vi "TestError.vi"() -> ()   [LabVIEW 2014, in "NISTErrorLib.lvlib"]
doc: "Use this template to build a producer/consumer design pattern with events to produce queue items. Use this design pattern instead of the User Interface Event Handler pattern for user interfaces when you want to execute code asynchronously in response to an event without slowing the user interface responsiveness."
uses:
  NISTErrorLib.lvlib
  <vilib>/Utility/error.llb/Error Cluster From Error Code.vi
  <vilib>/ErrorRing/Error Ring.xnode
panel:
  in  "btnLargeError":bool
  in  "btnLog":bool
  out "Log":string
  in  "btnMultiError":bool
  out "State":string
  in  "btnStateError":bool
  in  "btnUnhandled":bool
  in  "stop":bool
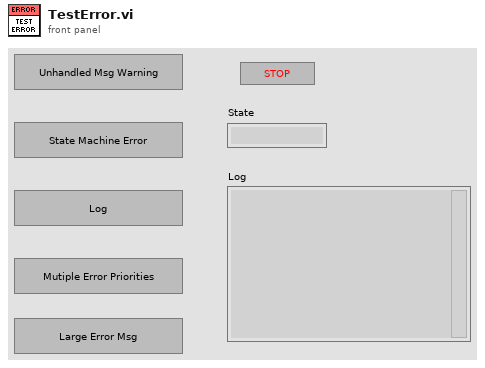
[diagram p1: front panel]
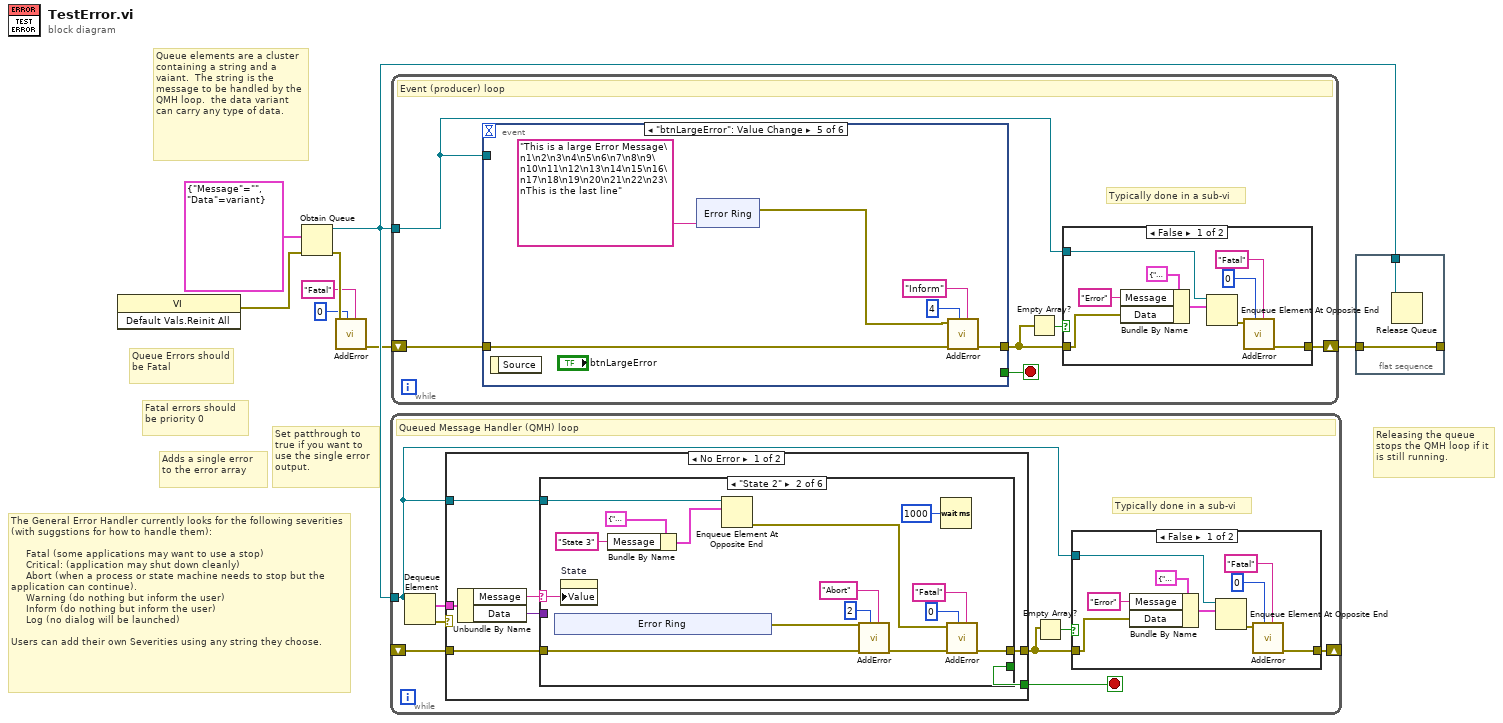
[diagram p0: block diagram]
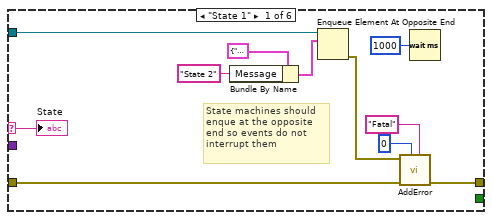
[diagram p3: hidden frame]
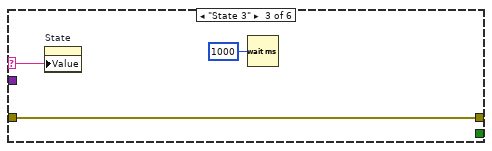
[diagram p4: hidden frame]
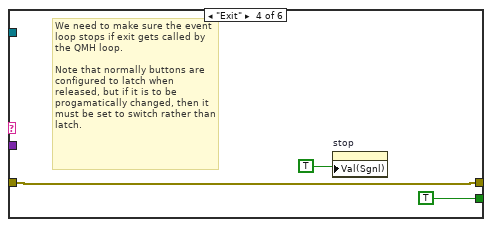
[diagram p5: hidden frame]
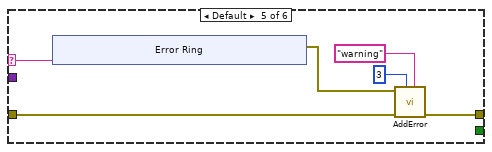
[diagram p6: hidden frame]
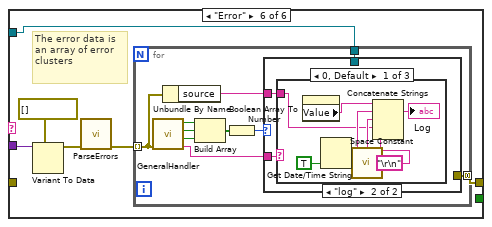
[diagram p7: hidden frame]
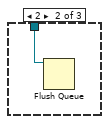
[diagram p9: hidden frame]
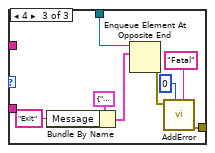
[diagram p10: hidden frame]
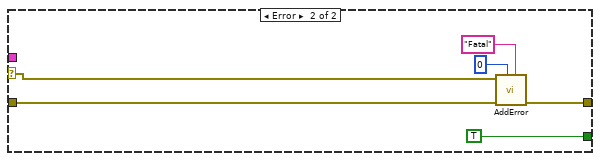
[diagram p11: hidden frame]
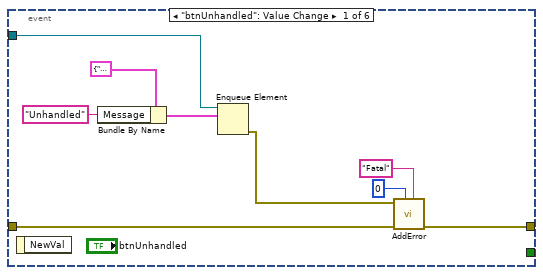
[diagram p13: hidden frame]
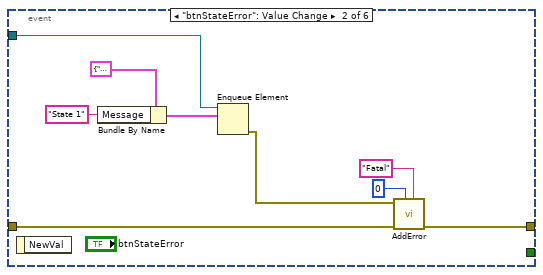
[diagram p14: hidden frame]
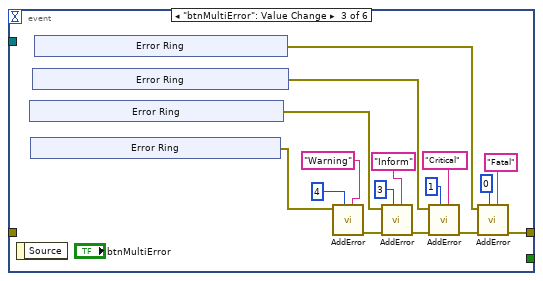
[diagram p15: hidden frame]
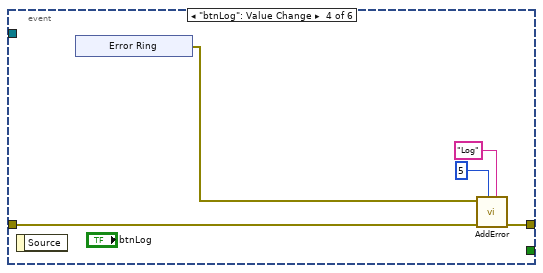
[diagram p16: hidden frame]
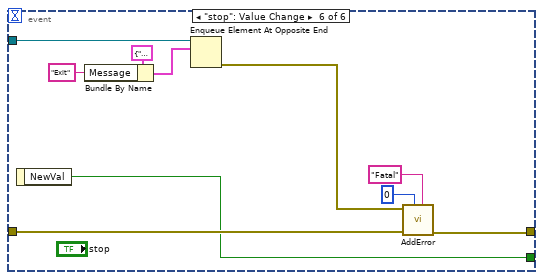
[diagram p17: hidden frame]
diagram:
  # "Set patthrough to\ntrue if you want to\nuse the single error \noutput."
  # "The General Error Handler currently looks for the following severities (with suggstions for how to handle them):\n\n     Fatal (some applications may want to use a stop)  \n     Critical: (application may shut down cleanly)\n     Abort (when a process or state machine needs to stop but the application can continue).\n     Warning (do nothing but inform the user)\n     Inform (do nothing but inform the user)\n     Log (no dialog will be launched)\n    \nUsers can add their own Severities using any string they choose."
  # "Adds a single error to the error array"
  # "Fatal errors should be priority 0"
  # "Queue elements are a cluster containing a string and a vaiant.  The string is the message to be handled by the QMH loop.  the data variant can carry any type of data."
  # "Queue Errors should be Fatal"
  # "Releasing the queue stops the QMH loop if it is still running."
  n1 = invoke class="VI" method="Default Vals.Reinit All"() -> (error out=w1:errorcluster)  [unwired: 3 in, 2 out]
  n2 = Obtain Queue(element data type=cluster{"Message":string, "Data":variant} {"Message"="", "Data"=variant}, error in (no error)=w1) -> (queue out=w8:refnum<queue>, error out=w6:errorcluster)  [unwired: 3 in, 1 out]
  n3 = call "AddError.vi"("Severity"="Fatal" ("String"), "Priority"=u8 0, "error in (no error)"=w6) -> ("ErrorArray"=w3:errorcluster[])  [unwired: 7 in, 1 out]
  n4 = while {
    tunnel: w8 -> [w11]
    shift-right: [w14] -> _
    shift-left: _ -> [w13]
    stop <- w15 stop-if-true
    # "Typically done in a sub-vi"
    # "Queued Message Handler (QMH) loop"
    n5 = Dequeue Element(queue=w11) -> (element=w12:cluster{"Message":string, "Data":variant}, error out=w16:errorcluster)  [unwired: 2 in, 2 out]
    n6 = case shown="No Error" w16 {
      selector: w16 -> [_ w120]
      tunnel: w12 -> [w33 _]
      tunnel: [w28 TRUE] -> w15
      tunnel: w13 -> [w31 w122]
      tunnel: [w30 w121] -> w10
      tunnel: w11 -> [w27 _]
      frame No Error {
        n7 = Unbundle By Name(w33) -> ("Message"=w32:string, "Data"=w29:variant)
        n8 = case shown="\"State 2\"" w32 {
          selector: w32 -> [w34 w51 w67 _ w76 _]
          tunnel: w31 -> [w36 w50 w66 w68 w75 _]
          tunnel: [w44 w59 w66 w68 w74 w84] -> w30
          tunnel: w29 -> [_ _ _ _ _ w86]
          tunnel: [_ _ _ TRUE _ _] -> w28
          tunnel: w27 -> [w41 w56 _ _ _ w85]
          frame "State 1" {
            # "State machines should enque at the opposite end so events do not interrupt them"
            n9 = Bundle By Name(cluster=cluster{"Message":string, "Data":variant} {"Message"="", "Data"=variant}, "Message"="State 2") -> (w38:cluster{"Message":string, "Data":variant})
            n10 = Enqueue Element At Opposite End(queue=w41, element=w38) -> (error out=w37:errorcluster)  [unwired: 2 in, 2 out]
            n11 = call "AddError.vi"("Severity"="Fatal" ("String"), "Priority"=u8 0, "ErrorArray"=w36, "error in (no error)"=w37) -> ("ErrorArray"=w44:errorcluster[])  [unwired: 6 in, 1 out]
            n12 = Wait (ms)(milliseconds to wait=u32 1000) -> ()  [unwired: 1 out]
            "State" <- w34
          }
          frame "State 2" {
            n13 = xnode "Error Ring"() -> ("error out"=w45:errorcluster)
            n14 = property on="State" class="Str"("Value"=w51) -> ()  [unwired: 2 in, 2 out]
            n15 = Bundle By Name(cluster=cluster{"Message":string, "Data":variant} {"Message"="", "Data"=variant}, "Message"="State 3") -> (w53:cluster{"Message":string, "Data":variant})
            n16 = Enqueue Element At Opposite End(queue=w56, element=w53) -> (error out=w46:errorcluster)  [unwired: 2 in, 2 out]
            n17 = call "AddError.vi"("Severity"="Abort" ("String"), "Priority"=u8 2, "ErrorArray"=w50, "error in (no error)"=w45) -> ("ErrorArray"=w49:errorcluster[])  [unwired: 6 in, 1 out]
            n18 = Wait (ms)(milliseconds to wait=u32 1000) -> ()  [unwired: 1 out]
            n19 = call "AddError.vi"("Severity"="Fatal" ("String"), "Priority"=u8 0, "ErrorArray"=w49, "error in (no error)"=w46) -> ("ErrorArray"=w59:errorcluster[])  [unwired: 6 in, 1 out]
          }
          frame "State 3" {
            n20 = property on="State" class="Str"("Value"=w67) -> ()  [unwired: 2 in, 2 out]
            n21 = Wait (ms)(milliseconds to wait=u32 1000) -> ()  [unwired: 1 out]
          }
          frame "Exit" {
            # "We need to make sure the event loop stops if exit gets called by the QMH loop.\n\nNote that normally buttons are configured to latch when released, but if it is to be progamatically changed, then it must be set to switch rather than latch."
            n22 = property on="stop" class="Bool (strict)"("Val(Sgnl)"=TRUE) -> ()  [unwired: 2 in, 2 out]
          }
          frame Default {
            n23 = xnode "Error Ring"("parameter 0"=w76) -> ("error out"=w73:errorcluster)
            n24 = call "AddError.vi"("Severity"="warning" ("String"), "Priority"=u8 3, "ErrorArray"=w75, "error in (no error)"=w73) -> ("ErrorArray"=w74:errorcluster[])  [unwired: 6 in, 1 out]
          }
          frame "Error" {
            # "The error data is an array of error clusters"
            n25 = Variant To Data(type=errorcluster[] [], Variant=w86) -> (data=w88:errorcluster[])  [unwired: 1 in, 1 out]
            n26 = call "ParseErrors.vi"("ErrorArray"=w88) -> ("ErrorArray"=w89:errorcluster[])  [unwired: 8 in, 2 out]
            n27 = for {
              tunnel: w89 -> [w91] mode=indexing
              tunnel: w85 -> [w94]
              tunnel: [w92] -> w84 mode=concatenating
              n28 = call "GeneralHandler.vi"("error in (no error)"=w91) -> ("Severity"=w93:string, "Stop"=w97:bool, "Abort"=w99:bool, "Continue"=w98:bool)  [unwired: 7 in]
              n29 = Unbundle By Name(w91) -> ("source"=w90:string)
              n30 = Build Array(w98, w99, w97) -> (w96:bool[])
              n31 = Boolean Array To Number(Boolean array=w96) -> (number=w95:u32)
              n32 = case shown="0, Default" w95 {
                tunnel: w94 -> [_ w109 w117]
                tunnel: w93 -> [w101 _ _]
                tunnel: [_ _ w113] -> w92
                tunnel: w90 -> [w100 _ _]
                frame 0, Default {
                  n33 = case shown="\"log\"" w101 {
                    tunnel: w100 -> [_ w103]
                    frame "False", Default {
                    }
                    frame "log" {
                      n34 = property on="Log" class="Str"() -> ("Value"=w107:string)  [unwired: 2 in, 2 out]
                      n35 = Get Date/Time String(want seconds? (F)=TRUE) -> (time string=w105:string)  [unwired: 2 in, 1 out]
                      n36 = call <vilib>:"Space Constant.vi"() -> ("String"=w104:string)
                      n37 = Concatenate Strings(w107, w105, w104, w103, "\r\n") -> (→"Log":string)
                    }
                  }
                }
                frame 2 {
                  n38 = Flush Queue(queue=w109) -> ()  [unwired: 1 in, 3 out]
                }
                frame 4 {
                  n39 = Bundle By Name(cluster=cluster{"Message":string, "Data":variant} {"Message"="", "Data"=variant}, "Message"="Exit") -> (w114:cluster{"Message":string, "Data":variant})
                  n40 = Enqueue Element At Opposite End(queue=w117, element=w114) -> (error out=w112:errorcluster)  [unwired: 2 in, 2 out]
                  n41 = call "AddError.vi"("Severity"="Fatal" ("String"), "Priority"=u8 0, "error in (no error)"=w112) -> ("ErrorArray"=w113:errorcluster[])  [unwired: 7 in, 1 out]
                }
              }
            }
          }
        }
      }
      frame Error {
        n42 = call "AddError.vi"("Severity"="Fatal" ("String"), "Priority"=u8 0, "ErrorArray"=w122, "error in (no error)"=w120) -> ("ErrorArray"=w121:errorcluster[])  [unwired: 6 in, 1 out]
      }
    }
    n43 = Empty Array?(array=w10) -> (empty?=w9:bool)
    n44 = case shown="False" w9 {
      tunnel: [w20 w26] -> w14
      tunnel: w10 -> [w24 w26]
      tunnel: w11 -> [w17 _]
      frame False {
        n45 = Bundle By Name(cluster=cluster{"Message":string, "Data":variant} {"Message"="", "Data"=variant}, "Message"="Error", "Data"=w24) -> (w23:cluster{"Message":string, "Data":variant})
        n46 = Enqueue Element At Opposite End(queue=w17, element=w23) -> (error out=w21:errorcluster)  [unwired: 2 in, 2 out]
        n47 = call "AddError.vi"("Severity"="Fatal" ("String"), "Priority"=u8 0, "error in (no error)"=w21) -> ("ErrorArray"=w20:errorcluster[])  [unwired: 7 in, 1 out]
      }
      frame True {
      }
    }
  }
  n48 = while {
    tunnel: w8 -> [w126]
    shift-right: [w127] -> w2
    shift-left: w3 -> [w128]
    stop <- w129 stop-if-true
    # "Typically done in a sub-vi"
    # "Event (producer) loop"
    n49 = event shown="[4] \"btnLargeError\": Value Change" {
      selector: _ -> [_ _ _ _ _ _]
      dyn-events: _ -> [_ _ _ _ _ _]
      timeout: _ -> [_ _ _ _ _ _]
      tunnel: w126 -> [w148 w157 _ _ _ w226]
      tunnel: [w146 w155 w173 w198 w208 w222] -> w124
      tunnel: [_ _ _ _ _ w217] -> w129
      tunnel: w128 -> [w147 w156 _ w197 w204 w220]
      event "btnUnhandled": Value Change {
        n50 = event-data() -> ()  [unwired: 1 in, 1 out]
        n51 = Bundle By Name(cluster=cluster{"Message":string, "Data":variant} {"Message"="", "Data"=variant}, "Message"="Unhandled") -> (w143:cluster{"Message":string, "Data":variant})
        n52 = Enqueue Element(queue=w148, element=w143) -> (error out=w145:errorcluster)  [unwired: 2 in, 2 out]
        n53 = call "AddError.vi"("Severity"="Fatal" ("String"), "Priority"=u8 0, "ErrorArray"=w147, "error in (no error)"=w145) -> ("ErrorArray"=w146:errorcluster[])  [unwired: 6 in, 1 out]
      }
      event "btnStateError": Value Change {
        n54 = event-data() -> ()  [unwired: 1 in, 1 out]
        n55 = Bundle By Name(cluster=cluster{"Message":string, "Data":variant} {"Message"="", "Data"=variant}, "Message"="State 1") -> (w152:cluster{"Message":string, "Data":variant})
        n56 = Enqueue Element(queue=w157, element=w152) -> (error out=w154:errorcluster)  [unwired: 2 in, 2 out]
        n57 = call "AddError.vi"("Severity"="Fatal" ("String"), "Priority"=u8 0, "ErrorArray"=w156, "error in (no error)"=w154) -> ("ErrorArray"=w155:errorcluster[])  [unwired: 6 in, 1 out]
      }
      event "btnMultiError": Value Change {
        n58 = event-data() -> ()  [unwired: 1 in, 1 out]
        n59 = xnode "Error Ring"() -> ("error out"=w163:errorcluster)
        n60 = xnode "Error Ring"() -> ("error out"=w160:errorcluster)
        n61 = xnode "Error Ring"() -> ("error out"=w166:errorcluster)
        n62 = xnode "Error Ring"() -> ("error out"=w169:errorcluster)
        n63 = call "AddError.vi"("Severity"="Warning" ("String"), "Priority"=u8 4, "error in (no error)"=w160) -> ("ErrorArray"=w170:errorcluster[])  [unwired: 7 in, 1 out]
        n64 = call "AddError.vi"("Severity"="Inform" ("String"), "Priority"=u8 3, "ErrorArray"=w170, "error in (no error)"=w163) -> ("ErrorArray"=w171:errorcluster[])  [unwired: 6 in, 1 out]
        n65 = call "AddError.vi"("Severity"="Critical" ("String"), "Priority"=u8 1, "ErrorArray"=w171, "error in (no error)"=w166) -> ("ErrorArray"=w172:errorcluster[])  [unwired: 6 in, 1 out]
        n66 = call "AddError.vi"("Severity"="Fatal" ("String"), "Priority"=u8 0, "ErrorArray"=w172, "error in (no error)"=w169) -> ("ErrorArray"=w173:errorcluster[])  [unwired: 6 in, 1 out]
      }
      event "btnLog": Value Change {
        n67 = event-data() -> ()  [unwired: 1 in, 1 out]
        n68 = xnode "Error Ring"() -> ("error out"=w196:errorcluster)
        n69 = call "AddError.vi"("Severity"="Log" ("String"), "Priority"=u8 5, "ErrorArray"=w197, "error in (no error)"=w196) -> ("ErrorArray"=w198:errorcluster[])  [unwired: 6 in, 1 out]
      }
      event "btnLargeError": Value Change {
        n70 = event-data() -> ()  [unwired: 1 in, 1 out]
        n71 = xnode "Error Ring"("parameter 0"="This is a large Error Message\n1\n2\n3\n4\n5\n6\n7\n8\n9\n10\n11\n12\n13\n14\n15\n16\n17\n18\n19\n20\n21\n22\n23\nThis is the last line") -> ("error out"=w205:errorcluster)
        n72 = call "AddError.vi"("Severity"="Inform", "Priority"=u8 4, "ErrorArray"=w204, "error in (no error)"=w205) -> ("ErrorArray"=w208:errorcluster[])  [unwired: 6 in, 1 out]
      }
      event "stop": Value Change {
        n73 = event-data() -> ("NewVal"=w217:bool)  [unwired: 1 in]
        n74 = Bundle By Name(cluster=cluster{"Message":string, "Data":variant} {"Message"="", "Data"=variant}, "Message"="Exit") -> (w223:cluster{"Message":string, "Data":variant})
        n75 = Enqueue Element At Opposite End(queue=w226, element=w223) -> (error out=w221:errorcluster)  [unwired: 2 in, 2 out]
        n76 = call "AddError.vi"("Severity"="Fatal" ("String"), "Priority"=u8 0, "ErrorArray"=w220, "error in (no error)"=w221) -> ("ErrorArray"=w222:errorcluster[])  [unwired: 6 in, 1 out]
      }
    }
    n77 = Empty Array?(array=w124) -> (empty?=w125:bool)
    n78 = case shown="False" w125 {
      tunnel: [w133 w139] -> w127
      tunnel: w124 -> [w137 w139]
      tunnel: w126 -> [w130 _]
      frame False {
        n79 = Bundle By Name(cluster=cluster{"Message":string, "Data":variant} {"Message"="", "Data"=variant}, "Message"="Error", "Data"=w137) -> (w136:cluster{"Message":string, "Data":variant})
        n80 = Enqueue Element At Opposite End(queue=w130, element=w136) -> (error out=w134:errorcluster)  [unwired: 2 in, 2 out]
        n81 = call "AddError.vi"("Severity"="Fatal" ("String"), "Priority"=u8 0, "error in (no error)"=w134) -> ("ErrorArray"=w133:errorcluster[])  [unwired: 7 in, 1 out]
      }
      frame True {
      }
    }
  }
  n82 = flat-sequence {
    tunnel: w8 -> [w228]
    tunnel: [w227] -> _
    tunnel: w2 -> [w227]
    frame #0 {
      n83 = Release Queue(queue=w228) -> ()  [unwired: 2 in, 3 out]
    }
  }
